vi "2D Look-Up Table (DBL).vi"(2 "LUT":dbl[][](array[numeric]) format="%.2f", 3 "y index (column)":dbl=0.1 format="%.2f", 4 "x index (row)":dbl=0.1 format="%.2f") -> (1 "output point":dbl format="%.2f")   [LabVIEW 2020, in "NI_AdvCtrl_nonlinear.lvlib"]
doc: "LabVIEW no longer supports this VI. You can obtain similar functionality by installing the LabVIEW Simulation Module.\n\nSearches for an element in a given 2D table that has a fractional x-index and y-index (interpolation)."
uses:
  <vilib>/addons/control/advanced/NI_AdvCtrl_nonlinear.lvlib
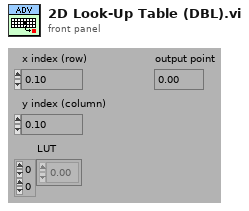
[diagram p1: front panel]
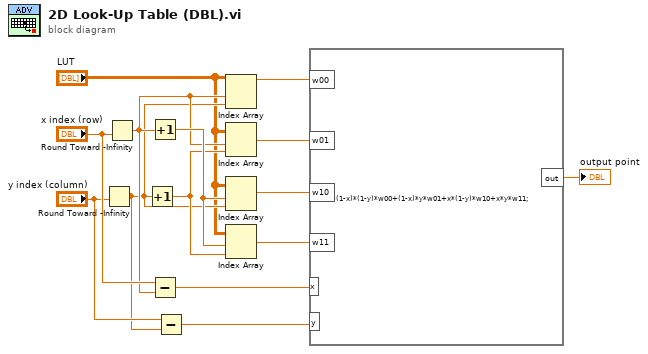
[diagram p0: block diagram]
diagram:
  n1 = Round Toward -Infinity(1:"y index (column)") -> (0:w7:dbl)
  n2 = Round Toward -Infinity(1:"x index (row)") -> (0:w10:dbl)
  n3 = Increment(x=w7) -> (x+1=w13:dbl)
  n4 = Increment(x=w10) -> (x+1=w14:dbl)
  n5 = Subtract(x="x index (row)", y=w10) -> (x-y=w9:dbl)
  n6 = Subtract(x="y index (column)", y=w7) -> (x-y=w6:dbl)
  n7 = Index Array(array="LUT", index (row)=w10, index (col)=w7) -> (element=w5:dbl)
  n8 = Index Array(array="LUT", index (row)=w10, index (col)=w13) -> (element=w4:dbl)
  n9 = Index Array(array="LUT", index (row)=w14, index (col)=w7) -> (element=w3:dbl)
  n10 = Index Array(array="LUT", index (row)=w14, index (col)=w13) -> (element=w2:dbl)
  n11 = formula code="out=(1-x)*(1-y)*w00+(1-x)*y*w01+x*(1-y)*w10+x*y*w11;"("w00"=w5, "w01"=w4, "w10"=w3, "w11"=w2, "x"=w9, "y"=w6) -> ("out"=→"output point":dbl)
